vi "Read Serialization Binder.vi"(8 "error in (no error)":errorcluster, 11 "Flatten To JSON Object in":refnum<class "Generic Object Serializer.lvclass">) -> (0 "error out":errorcluster, 2 "Serialization Binder":refnum<class "Serialization Binder.lvclass">, 3 "Flatten To JSON Object out":refnum<class "Generic Object Serializer.lvclass">)   [LabVIEW 2017, in "Generic Object Serializer.lvclass"]
doc: "Returns the serialization binder or <B>Default Serialization Binder</B> if no serialization binder is specified."
uses:
  Generic Object Serializer/Generic Object Serializer.lvclass
  Serialization Binder/Serialization Binder.lvclass
  Generic Object Serializer/Generic Object Serializer.lvclass/Generic Object Serializer.ctl
  Default Serialization Binder/Default Serialization Binder.lvclass
  C:/Users/de200256/Code/logmanoriginal/jsontext-object-serialization/Serialization Binder/Serialization Binder.lvclass
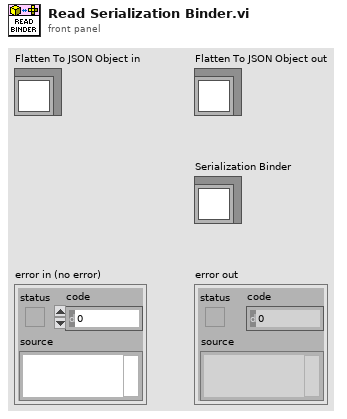
[diagram p1: front panel]
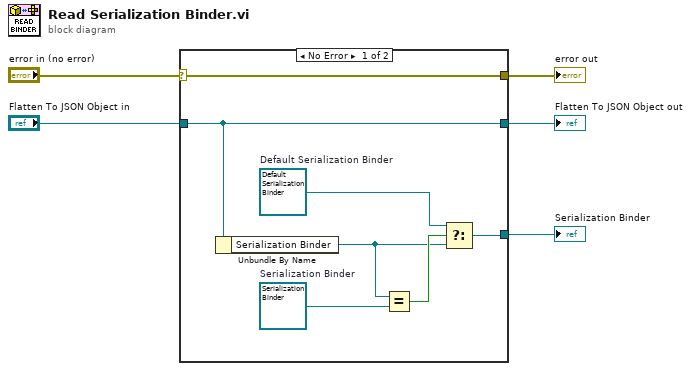
[diagram p0: block diagram]
diagram:
  n1 = case shown="No Error" "error in (no error)" {
    selector: "error in (no error)" -> [w12 w13]
    tunnel: [w12 w13] -> w4
    tunnel: [w11 w14] -> w2
    tunnel: "Flatten To JSON Object in" -> [w11 w14]
    tunnel: [w7 _] -> w1
    frame No Error {
      w6 = refnum<class "Default Serialization Binder.lvclass"> refnum  # Default Serialization Binder
      w10 = refnum<class "Serialization Binder.lvclass"> refnum  # Serialization Binder
      n2 = Unbundle By Name(w11) -> ("Serialization Binder"=w8:refnum<class "Serialization Binder.lvclass">)
      n3 = Equal?(x=w8, y=w10) -> (x = y?=w9:bool)
      n4 = Select(t=w6, s=w9, f=w8) -> (s? t:f=w7:refnum<class "Serialization Binder.lvclass">)
    }
    frame Error {
    }
  }
  "error out" <- w4
  "Flatten To JSON Object out" <- w2
  "Serialization Binder" <- w1
